vi "RH (T) Probe Global Var.vi"() -> ()   [LabVIEW 2011]
panel:
  in  "RH (T) Probes":dbl
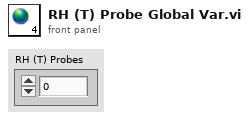
[diagram p1: front panel]
diagram:
